vi "DP-Insert Notes.vi"(0 "path":path, 7 "Notes":string, 11 "error in (no error)":errorcluster) -> (15 "error out":errorcluster)   [LabVIEW 2020]
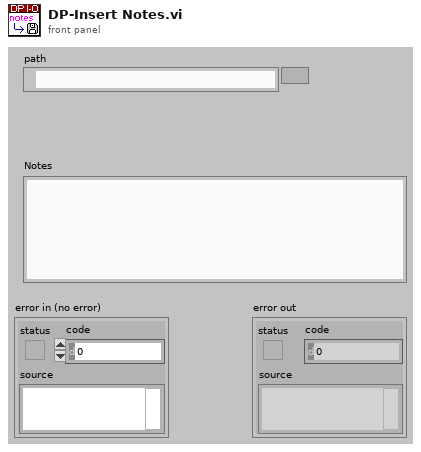
[diagram p1: front panel]
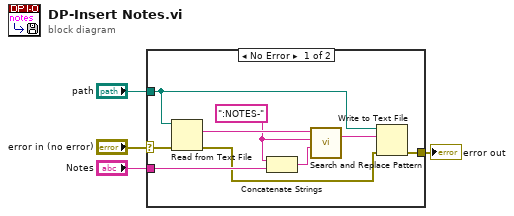
[diagram p0: block diagram]
diagram:
  n1 = case shown="No Error" "error in (no error)" {
    selector: "error in (no error)" -> [w5 w14]
    tunnel: "Notes" -> [w11 _]
    tunnel: "path" -> [w9 _]
    tunnel: [w6 w14] -> w2
    frame No Error {
      w12 = ":NOTES-" ("regular expression (\"\")")
      n2 = Read from Text File(file (use dialog)=w9, error in=w5) -> (text=w13:string, error out=w7:errorcluster)  [unwired: 2 in, 2 out]
      n3 = Concatenate Strings(w12, w11) -> (w10:string)
      n4 = call <vilib>:"Search and Replace Pattern.vi"("string"=w13, "regular expression (\"\")"=w12, "replace string (\"\")"=w10) -> ("result string"=w8:string)  [unwired: 2 in, 1 out]
      n5 = Write to Text File(file (use dialog)=w9, text=w8, error in=w7) -> (error out=w6:errorcluster)  [unwired: 1 in, 2 out]
    }
    frame Error {
    }
  }
  "error out" <- w2
